vi "DefaultFromIni.vi"(8 "error in (no error)":errorcluster, 11 "MyPluginsBase in":refnum<class "Simulation.lvclass">) -> (0 "error out":errorcluster, 3 "MyPluginsBase out":refnum<class "Simulation.lvclass">)   [LabVIEW 2018, in "DigitizerPlugins.lvlib" / "Simulation.lvclass"]
uses:
  Simulation.lvclass
  C:/Program Files/National Instruments/LabVIEW 2018/user.lib/NIST/BaseClasses/BasePlugin_class/BasePlugin.lvclass
  <userlib>/NIST/BaseClasses/BasePlugin_class/BasePlugin.lvclass/BasePlugin.ctl
  FGen/MemberClasses/FunctionBaseClass/FunctionBase.lvclass
  Simulation.lvclass/Simulation.ctl
  <userlib>/NIST/BaseClasses/BasePlugin_class/Accessors/Read PluginIniFilePath.vi
  Accessors/Write FunctionIniFilePath.vi
  Accessors/Write Function.vi
  <vilib>/Utility/error.llb/Error Cluster From Error Code.vi
  DigitizerBaseClass/DigitizerBase.lvclass
  <vilib>/ErrorRing/Error Ring.xnode
  <vilib>/Utility/config.llb/NI_LVConfig.lvlib
  <userlib>/NIST/BaseClasses/Object_class/BaseObject.lvclass
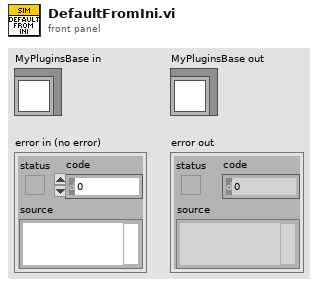
[diagram p1: front panel]
types:
  T1 = typedef "NI_LVConfig.lvlib/Config Data RefNum.ctl" = refnum<k1>
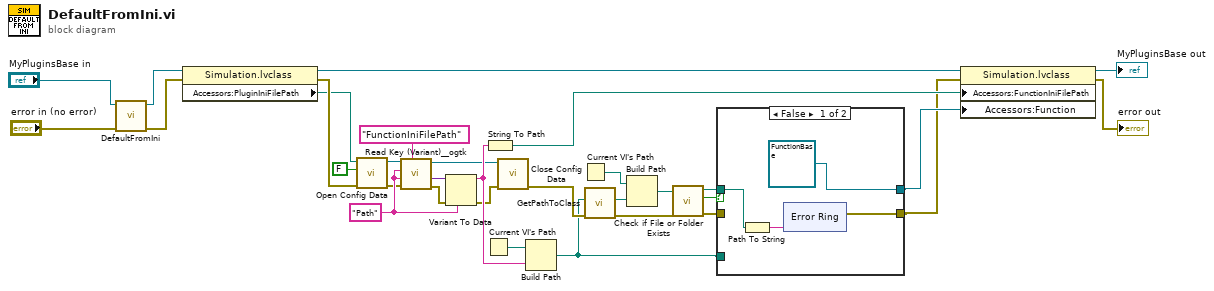
[diagram p0: block diagram]
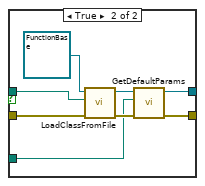
[diagram p2: hidden frame]
diagram:
  w20 = "Path" ("key (optional)")
  n1 = call-parent "DefaultFromIni.vi"("error in (no error)"="error in (no error)", "MyPluginsBase in"="MyPluginsBase in") -> ("error out"=w13:errorcluster, "MyPluginsBase out"=w14:refnum<class "Simulation.lvclass">)  [unwired: 8 in]
  n2 = property class="Simulation.lvclass"(reference=w14, error in=w13) -> (reference out=w10:refnum<class "Simulation.lvclass">, error out=w12:errorcluster, "Accessors:PluginIniFilePath"=w11:path)
  n3 = call <vilib>:"Open Config Data.vi"("error in (no error)"=w12, "create file if necessary (T)"=FALSE, "configuration file path"=w11) -> ("error out"=w16:errorcluster, "refnum"=w30:T1)  [unwired: 6 in, 1 out]
  n4 = call <userlib>:"Read Key (Variant)__ogtk.vi"("section"="FunctionIniFilePath", "error in (no error)"=w16, "type"=w20, "key (optional)"=w20, "refnum"=w30) -> ("error out"=w18:errorcluster, "key-value"=w19:variant, "refnum out"=w21:T1)  [unwired: 3 in, 1 out]
  n5 = Variant To Data(error in=w18, type=w20, Variant=w19) -> (data=w29:string, error out=w22:errorcluster)
  n6 = Current VI's Path() -> (path=w28:path)
  n7 = String To Path(string=w29) -> (path=w9:path)
  n8 = call <vilib>:"Close Config Data.vi"("error in (no error)"=w22, "refnum"=w21) -> ("error out"=w23:errorcluster)  [unwired: 8 in, 1 out]
  n9 = Build Path(base path=w28, name or relative path=w29) -> (appended path=w7:path)
  n10 = Current VI's Path() -> (path=w24:path)
  n11 = call <userlib>:"GetPathToClass.vi"("error in (no error)"=w23, "configuration file path"=w7) -> ("error IO"=w27:errorcluster, "PathToClass"=w25:path)  [unwired: 8 in]
  n12 = Build Path(base path=w24, name or relative path=w25) -> (appended path=w26:path)
  n13 = call <vilib>:"Check if File or Folder Exists.vi"("error in (no error)"=w27, "path"=w26) -> ("error out"=w6:errorcluster, "file or folder exists?"=w1:bool, "dup path"=w8:path)  [unwired: 7 in]
  n14 = case shown="False" w1 {
    tunnel: [w35 w46] -> w4
    tunnel: w6 -> [_ w51]
    tunnel: w8 -> [w34 w50]
    tunnel: w7 -> [_ w44]
    tunnel: [refnum<class "FunctionBase.lvclass"> refnum ("Functions.lvlib:FunctionBase.lvclass") w45] -> w5
    frame False {
      n15 = Path To String(path=w34) -> (string=w36:string)
      n16 = xnode "Error Ring"("parameter 0"=w36) -> ("error out"=w35:errorcluster)
    }
    frame True {
      n17 = call-dynamic "LoadClassFromFile.vi"("error in (no error)"=w51, "class path"=w50, "reference in"=refnum<class "FunctionBase.lvclass"> refnum ("Functions.lvlib:FunctionBase.lvclass")) -> ("error out"=w48:errorcluster, "reference out"=w47:refnum<class "FunctionBase.lvclass">)  [unwired: 7 in]
      n18 = call-dynamic "GetDefaultParams.vi"("error in (no error)"=w48, "Path"=w44, "FunctionBase in"=w47) -> ("error out"=w46:errorcluster, "FunctionBase out"=w45:refnum<class "FunctionBase.lvclass">)  [unwired: 7 in]
    }
  }
  n19 = property class="Simulation.lvclass"(reference=w10, error in=w4, "Accessors:FunctionIniFilePath"=w9, "Accessors:Function"=w5) -> (reference out=→"MyPluginsBase out":refnum<class "Simulation.lvclass">, error out=→"error out":errorcluster)
